vi "Oclaro_FB_INJ_Anritsu.vi"() -> ()   [LabVIEW 2014]
doc: "Use this template to measure or generate signals using the DAQ Assistant Express VI and NI-DAQmx. Double click the DAQ Assistant Express VI to launch a configuration wizard which steps you through configuring a measurement or generation.\n\nNote: You must have an NI-DAQmx compatible device installed to use this Express VI. Refer to the DAQ Quick Start Guide for NI-DAQ 7.0 for a list of compatible devices."
uses:
  Instance           8 18Saved   INJ FB Map .vi
  <instrlib>/Tektronix 7000 Series/Public/Data/Read (Single Waveform).vi
  <instrlib>/Tektronix 7000 Series/Tektronix 7000 Series.lvlib
panel:
  in  "Capture OSA?":bool=TRUE
  in  "Scope Model":string="Tektronix MSO 71254"
  in  "OSA Model":string="Anritsu MS9710C"
  out "Current Source":string="PROFILE-ITC510"
  in  "Resistance (k Ohms)":dbl=10.0
  in  "Time Series Length":dbl=500000.0
  in  "OSA Address":refnum<visa-resource-name>="GPIB0::8::INSTR"
  in  "file path":path=path "Z:/Toomey/Experimental Data/Bangor DFB/2015-07-10/Run01/Data"
  in  "Tek Scope Address":refnum<visa-resource-name>="GPIB0::4::INSTR"
  out "Start time":timestamp=timestamp(3519349015.1862907 s since 1904-01-01)
  in  "Current Source Address":refnum<visa-resource-name>="GPIB0::10::INSTR"
  in  "Channel (0: Channel 1)":u16(ring) format="%#_5f" items=["Channel 1", "Channel 2", "Channel 3", "Channel 4", "Math 1", "Math 2", "Math 3", "Math 4", "Reference 1", "Reference 2", "Reference 3", "Reference 4"]
  out "Current FB":dbl=0.9
  out "Current INJ":dbl=80.0
  in  "Initial Current (mA)":dbl=25.0
  in  "Step Size (mA)":dbl=0.5
  in  "Max Current (mA)":dbl=80.0
  in  "AOM Step":dbl=0.005
  in  "AOM Finish":dbl=0.9
  in  "AOM Start":dbl=0.1
  out "Total Time (hrs)":dbl=47.11827769252989
  out "Finish time":timestamp=timestamp(3519518640.985984 s since 1904-01-01)
  out "INJ (%)":dbl=99.09909909909909
  out "FB (%)":dbl=99.37888198757764
  in  "Time to wait for TEC (sec)":dbl=15.0 caption="Delay Time (s)"
  # "Settings"
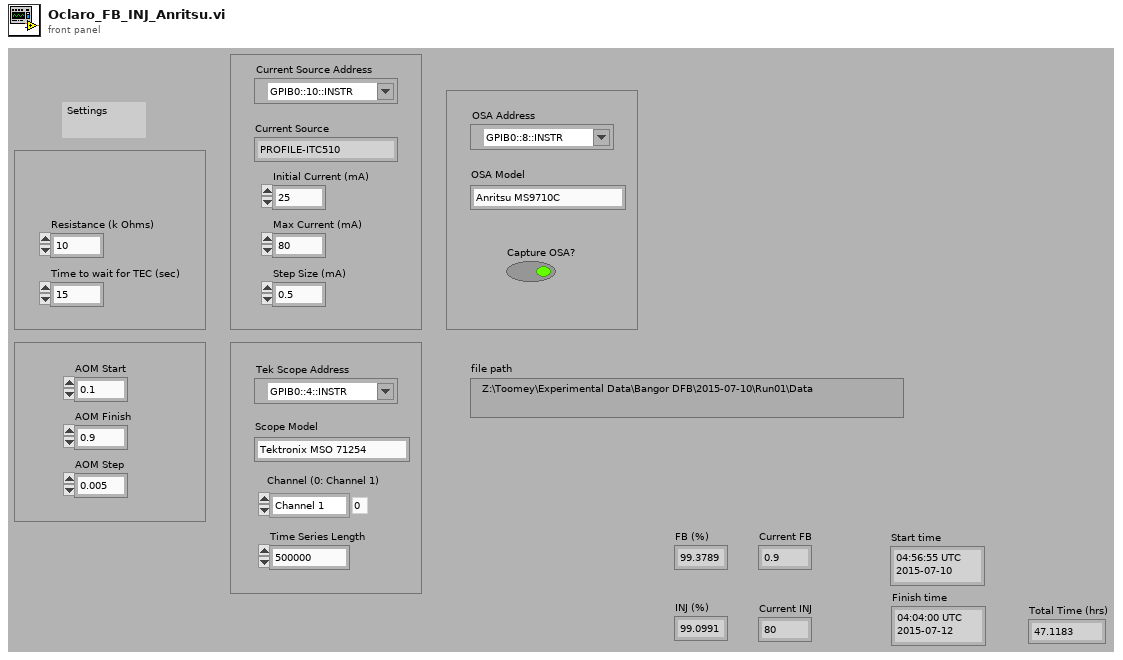
[diagram p1: front panel]
types:
  T1 = cluster{"Start Wavelength(nm)":dbl, "Stop Wavelength(nm)":dbl, "Sampling Points":i32}
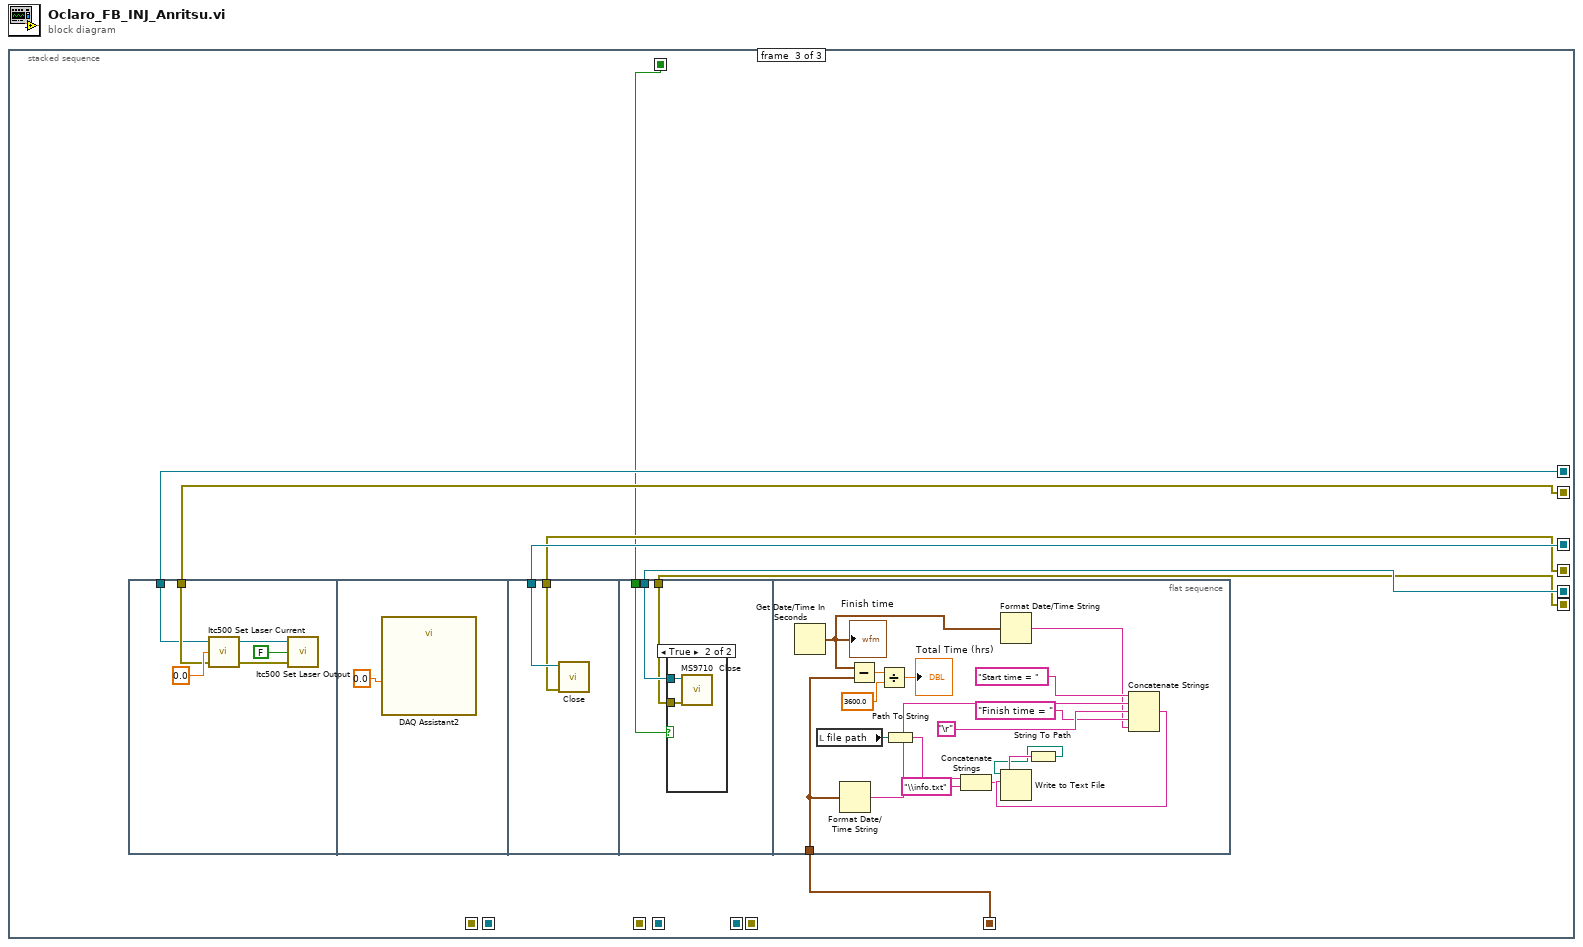
[diagram p0: block diagram]
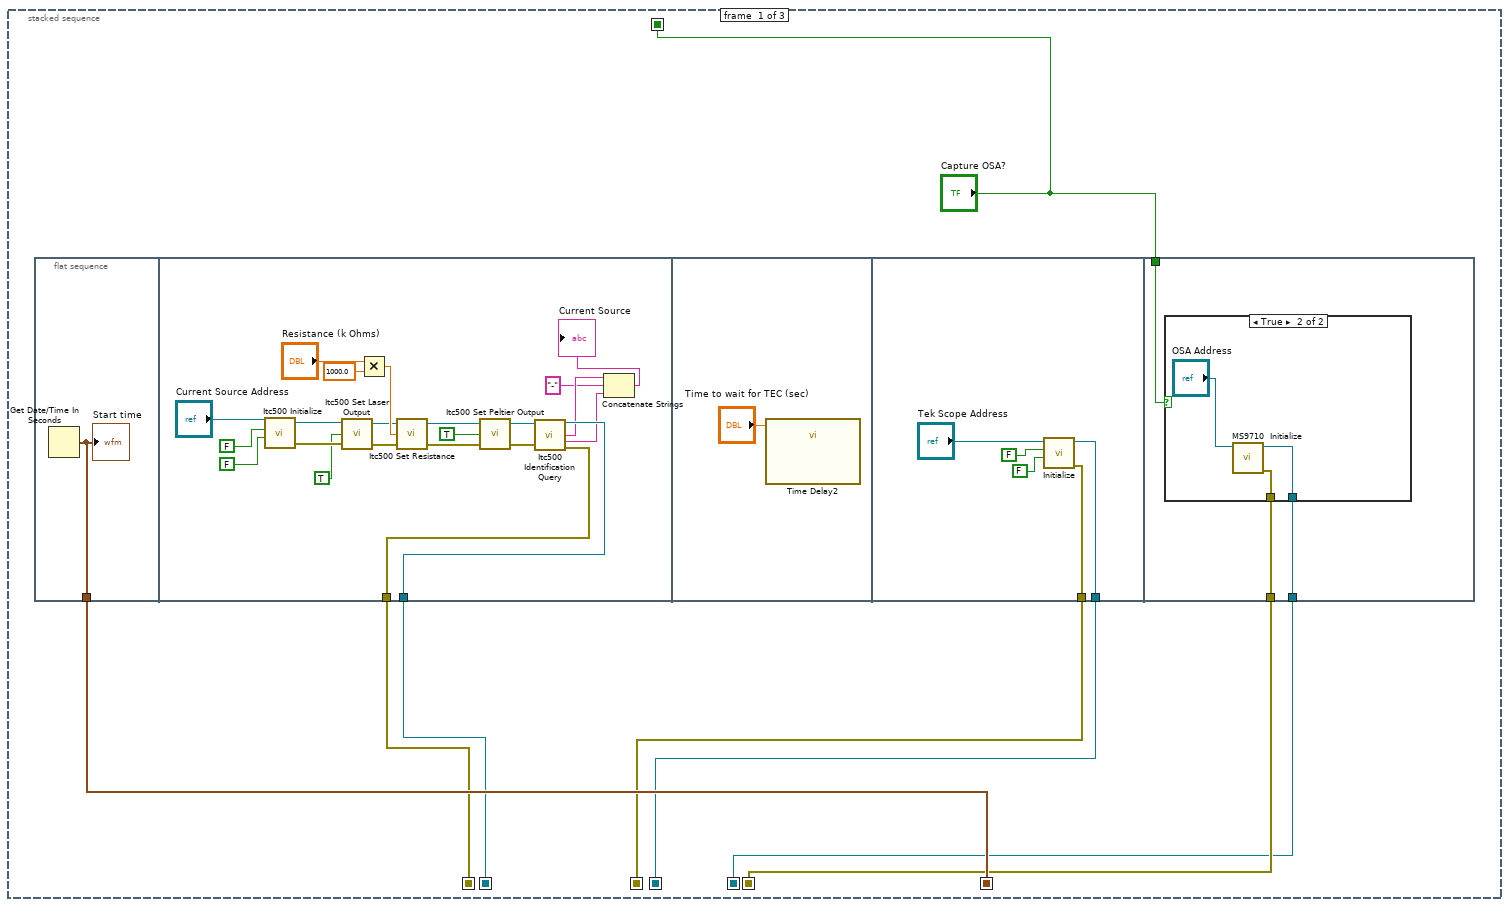
[diagram p2: hidden frame]
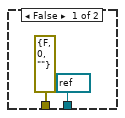
[diagram p3: hidden frame]
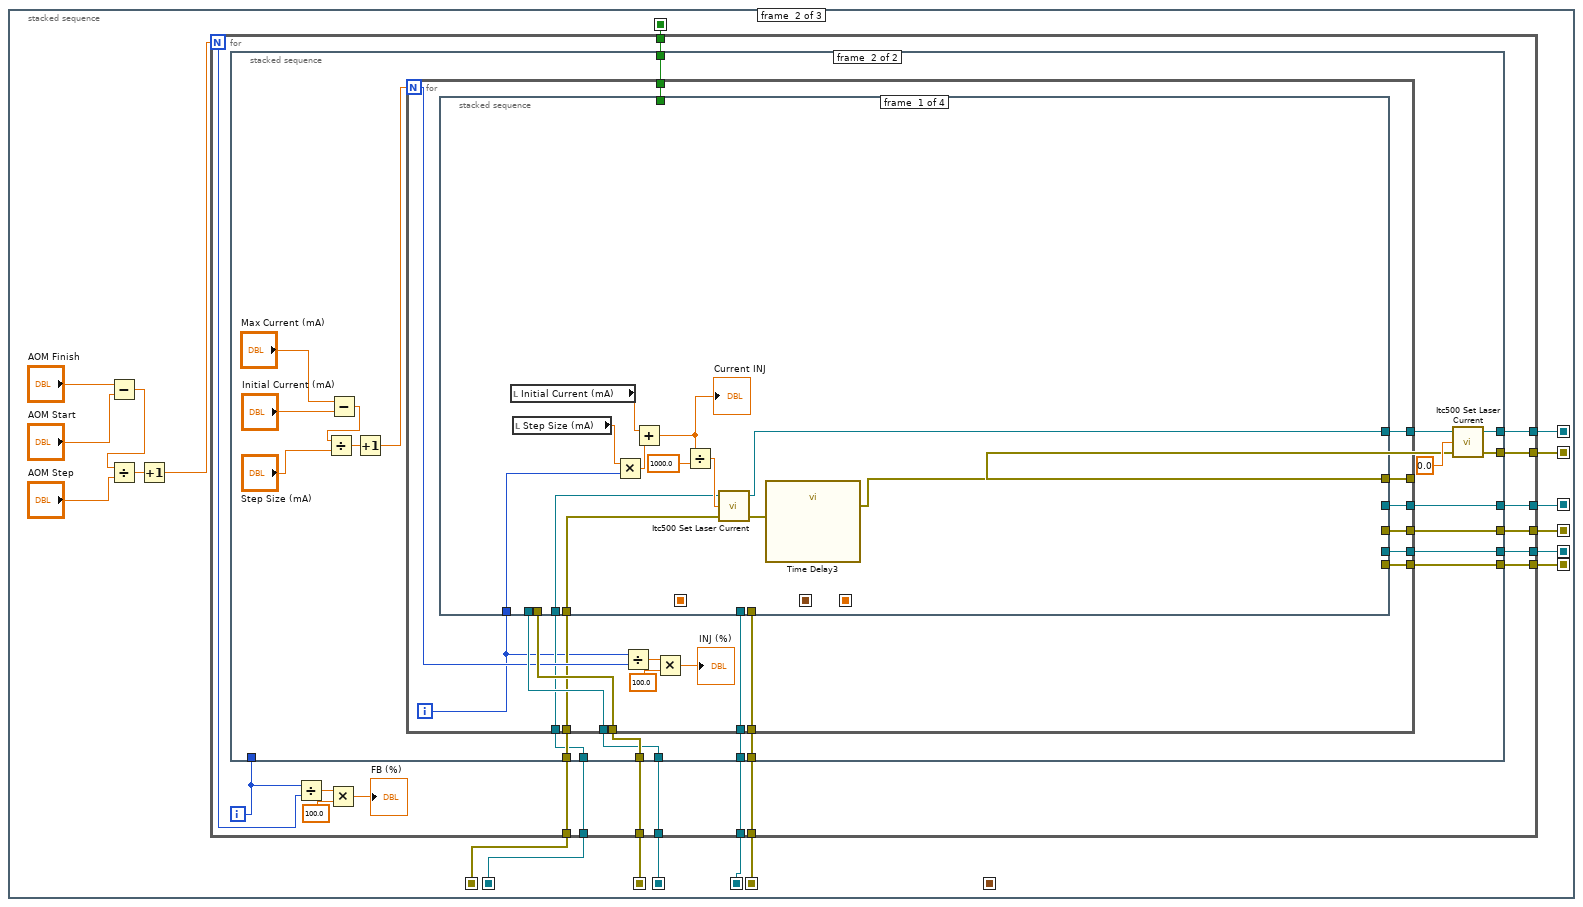
[diagram p4: hidden frame]
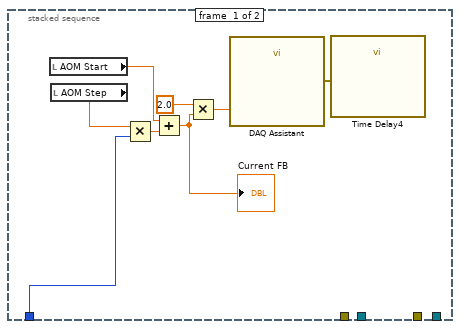
[diagram p5: hidden frame]
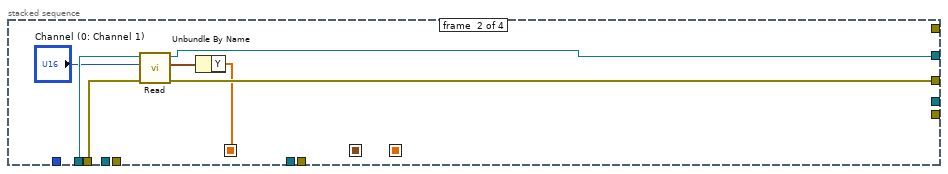
[diagram p6: hidden frame]
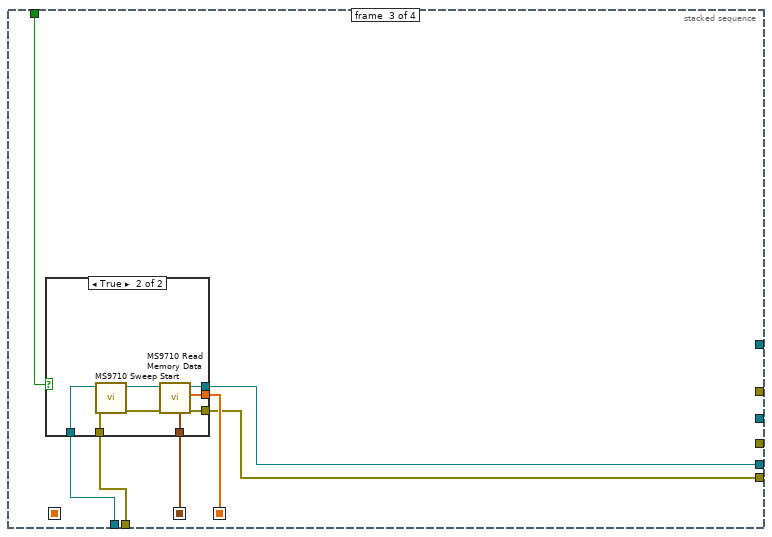
[diagram p7: hidden frame]
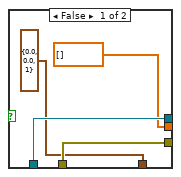
[diagram p8: hidden frame]
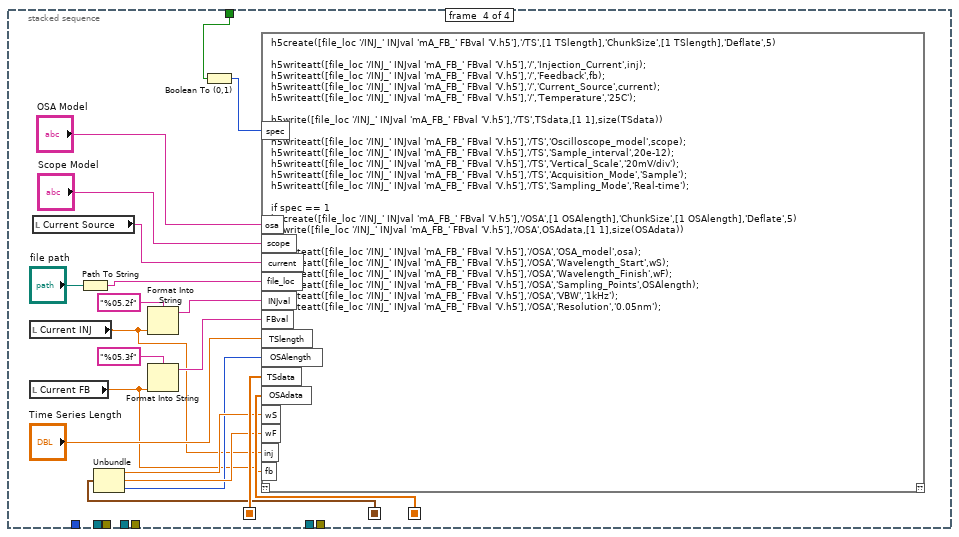
[diagram p9: hidden frame]
diagram:
  n1 = stacked-sequence {
    seq-local: [w5 _ _] -> [_ w62 _]
    seq-local: [w4 _ _] -> [_ w61 _]
    seq-local: [_ w60 _] -> [_ _ w195]
    seq-local: [_ w59 _] -> [_ _ w196]
    seq-local: [w8 _ _] -> [_ _ w192]
    seq-local: [_ w57 _] -> [_ _ w194]
    seq-local: [_ w56 _] -> [_ _ w193]
    seq-local: [w6 _ _] -> [_ w51 _]
    seq-local: [w7 _ _] -> [_ w52 _]
    seq-local: [w2 _ _] -> [_ w50 _]
    seq-local: [w3 _ _] -> [_ w49 _]
    seq-local: [_ w48 _] -> [_ _ w191]
    seq-local: [_ w47 _] -> [_ _ w190]
    seq-local: ["Capture OSA?" _ _] -> [_ w46 w189]
    frame #0 {
      n2 = flat-sequence {
        tunnel: [w9] -> w8
        tunnel: [w15] -> w7
        tunnel: [w14] -> w6
        tunnel: [w34] -> w5
        tunnel: [w33] -> w4
        tunnel: [w40] -> w3
        tunnel: [w39] -> w2
        tunnel: "Capture OSA?" -> [w38]
        frame #0 {
          n3 = Get Date/Time In Seconds() -> (seconds since 1Jan1904=w9:timestamp)
          "Start time" <- w9
        }
        frame #1 {
          n4 = call <instrlib>:"Itc500 Initialize.vi"("reset device"=FALSE, "id query"=FALSE, "resource name"="Current Source Address") -> ("error out"=w31:errorcluster, "instrument handle"=w30:refnum<visa-resource-name>)  [unwired: 1 in, 1 out]
          n5 = call <instrlib>:"Itc500 Set Laser Output.vi"("error in (no error)"=w31, "output"=TRUE, "instrument handle"=w30) -> ("error out"=w19:errorcluster, "instrument handle out"=w18:refnum<visa-resource-name>)  [unwired: 1 out]
          n6 = Multiply(x="Resistance (k Ohms)", y=1000.0) -> (x*y=w25:dbl)
          n7 = call <instrlib>:"Itc500 Set Resistance.vi"("error in (no error)"=w19, "resistance"=w25, "instrument handle"=w18) -> ("error out"=w21:errorcluster, "instrument handle out"=w20:refnum<visa-resource-name>)  [unwired: 1 out]
          n8 = call <instrlib>:"Itc500 Set Peltier Output.vi"("error in (no error)"=w21, "output"=TRUE, "instrument handle"=w20) -> ("error out"=w17:errorcluster, "instrument handle out"=w16:refnum<visa-resource-name>)  [unwired: 1 out]
          n9 = call <instrlib>:"Itc500 Identification Query.vi"("instrument handle"=w16, "error in (no error)"=w17) -> ("instrument handle out"=w14:refnum<visa-resource-name>, "manufacturer name"=w13:string, "instrument name"=w12:string, "error out"=w15:errorcluster)  [unwired: 7 in, 3 out]
          n10 = Concatenate Strings(w13, "-" ("string"), w12) -> (→"Current Source":string)
        }
        frame #2 {
          n11 = call "Time Delay2"("Delay Time (s)"="Time to wait for TEC (sec)") -> ()  [unwired: 10 in, 1 out]
        }
        frame #3 {
          n12 = call <instrlib>:"Initialize.vi"("Reset? ( Yes)"=FALSE ("Reset (T: Reset)"), "ID Query? ( Yes)"=FALSE ("Reset (T: Reset)"), "VISA resource name"="Tek Scope Address") -> ("error out"=w34:errorcluster, "VISA resource name out"=w33:refnum<visa-resource-name>)  [unwired: 7 in]
        }
        frame #4 {
          n13 = case shown="True" w38 {
            tunnel: [errorcluster {"status"=FALSE, "code"=0, "source"=""} ("error out") w44] -> w40
            tunnel: [refnum<visa-resource-name> refnum ("instr handle out") w43] -> w39
            frame False {
            }
            frame True {
              n14 = call <instrlib>:"MS9710  Initialize.vi"("VISA in"="OSA Address") -> ("error out"=w44:errorcluster, "instr handle out"=w43:refnum<visa-resource-name>)  [unwired: 9 in]
            }
          }
        }
      }
    }
    frame #1 {
      n15 = Subtract(x="AOM Finish", y="AOM Start") -> (x-y=w63:dbl)
      n16 = Divide(x=w63, y="AOM Step") -> (x/y=w64:dbl)
      n17 = Increment(x=w64) -> (x+1=w58:dbl)
      n18 = for {
        N: w58 -> [w75]
        tunnel: w51 -> [w82]
        tunnel: w52 -> [w81]
        tunnel: w62 -> [w80]
        tunnel: w61 -> [w79]
        tunnel: [w78] -> w60
        tunnel: [w77] -> w59
        tunnel: [w71] -> w57
        tunnel: [w70] -> w56
        tunnel: w50 -> [w69]
        tunnel: w49 -> [w68]
        tunnel: [w67] -> w48
        tunnel: [w66] -> w47
        tunnel: w46 -> [w65]
        i -> [w76]
        n19 = stacked-sequence {
          tunnel: w82 -> [_ w100]
          tunnel: w81 -> [_ w101]
          tunnel: w76 -> [w90 _]
          tunnel: w80 -> [_ w112]
          tunnel: w79 -> [_ w111]
          tunnel: [_ w97] -> w78
          tunnel: [_ w96] -> w77
          tunnel: [_ w107] -> w71
          tunnel: [_ w106] -> w70
          tunnel: w69 -> [_ w95]
          tunnel: w68 -> [_ w94]
          tunnel: [_ w93] -> w67
          tunnel: [_ w92] -> w66
          tunnel: w65 -> [_ w91]
          frame #0 {
            n20 = local read "AOM Start"() -> (w85:dbl)
            n21 = local read "AOM Step"() -> (w86:dbl)
            n22 = Multiply(x=w86, y=w90) -> (x*y=w89:dbl)
            n23 = Add(x=w85, y=w89) -> (x+y=w88:dbl)
            "Current FB" <- w88
            n24 = Multiply(x=2.0, y=w88) -> (x*y=w87:dbl)
            n25 = call "DAQ Assistant"("data"=w87) -> ("error out"=w84:errorcluster)  [unwired: 17 in, 1 out]
            n26 = call "Time Delay4"("error in (no error)"=w84) -> ()  [unwired: 10 in, 1 out]
          }
          frame #1 {
            n27 = Subtract(x="Max Current (mA)", y="Initial Current (mA)") -> (x-y=w109:dbl)
            n28 = Divide(x=w109, y="Step Size (mA)") -> (x/y=w110:dbl)
            n29 = Increment(x=w110) -> (x+1=w108:dbl)
            n30 = for {
              N: w108 -> [w124]
              tunnel: [w130] -> w99
              tunnel: w112 -> [w129]
              tunnel: w111 -> [w128]
              tunnel: [w123] -> w107
              tunnel: [w122] -> w106
              tunnel: w101 -> [w121]
              tunnel: w100 -> [w120]
              tunnel: [w119] -> w98
              tunnel: w95 -> [w117]
              tunnel: w94 -> [w116]
              tunnel: [w115] -> w93
              tunnel: [w114] -> w92
              tunnel: w91 -> [w113]
              i -> [w118]
              n31 = stacked-sequence {
                seq-local: [_ w143 _ _] -> [_ _ _ w186]
                seq-local: [_ _ w156 _] -> [_ _ _ w185]
                seq-local: [_ _ w155 _] -> [_ _ _ w184]
                tunnel: w118 -> [w136 _ _ _]
                tunnel: [w133 _ _ _] -> w130
                tunnel: w129 -> [_ w148 _ _]
                tunnel: w128 -> [_ w149 _ _]
                tunnel: [_ w146 _ _] -> w123
                tunnel: [_ w144 _ _] -> w122
                tunnel: w121 -> [w135 _ _ _]
                tunnel: w120 -> [w134 _ _ _]
                tunnel: [w132 _ _ _] -> w119
                tunnel: w117 -> [_ _ w154 _]
                tunnel: w116 -> [_ _ w153 _]
                tunnel: [_ _ w152 _] -> w115
                tunnel: [_ _ w151 _] -> w114
                tunnel: w113 -> [_ _ w150 w170]
                frame #0 {
                  n32 = local read "Initial Current (mA)"() -> (w138:dbl)
                  n33 = local read "Step Size (mA)"() -> (w137:dbl)
                  n34 = Multiply(x=w137, y=w136) -> (x*y=w141:dbl)
                  n35 = Add(x=w138, y=w141) -> (x+y=w131:dbl)
                  "Current INJ" <- w131
                  n36 = Divide(x=w131, y=1000.0) -> (x/y=w139:dbl)
                  n37 = call <instrlib>:"Itc500 Set Laser Current.vi"("error in (no error)"=w135, "current"=w139, "instrument handle"=w134) -> ("error out"=w140:errorcluster, "instrument handle out"=w132:refnum<visa-resource-name>)  [unwired: 1 out]
                  n38 = call "Time Delay3"("error in (no error)"=w140) -> ("error out"=w133:errorcluster)  [unwired: 10 in]
                }
                frame #1 {
                  n39 = call-poly <instrlib>:"Read.vi"("error in (no error)"=w148, "Channel (0: Channel 1)"="Channel (0: Channel 1)", "VISA resource name"=w149) -> ("error out"=w144:errorcluster, "Waveform Data"=w147:waveform(dbl), "VISA resource name out"=w146:refnum<visa-resource-name>)  [unwired: 6 in]
                  n40 = Unbundle By Name(w147) -> ("Y"=w143:dbl[])
                }
                frame #2 {
                  n41 = case shown="True" w150 {
                    tunnel: [dbl[] [] ("Data") w166] -> w156
                    tunnel: [T1 {"Start Wavelength(nm)"=0.0, "Stop Wavelength(nm)"=0.0, "Sampling Points"=1} ("Condition Data") w165] -> w155
                    tunnel: w154 -> [w159 w164]
                    tunnel: w153 -> [w160 w163]
                    tunnel: [w159 w162] -> w152
                    tunnel: [w160 w161] -> w151
                    frame False {
                    }
                    frame True {
                      n42 = call <instrlib>:"MS9710 Sweep Start.vi"("error in (no error)"=w163, "instr handle in"=w164) -> ("error out"=w168:errorcluster, "instr handle out"=w167:refnum<visa-resource-name>)  [unwired: 8 in]
                      n43 = call <instrlib>:"MS9710 Read Memory Data.vi"("error in (no error)"=w168, "instr handle in"=w167) -> ("error out"=w161:errorcluster, "Data"=w166:dbl[], "instr handle out"=w162:refnum<visa-resource-name>, "Condition Data"=w165:T1)  [unwired: 5 in, 1 out]
                    }
                  }
                }
                frame #3 {
                  n44 = local read "Current INJ"() -> (w171:dbl)
                  n45 = local read "Current FB"() -> (w172:dbl)
                  n46 = local read "Current Source"() -> (w175:string)
                  n47 = Path To String(path="file path") -> (string=w188:string)
                  n48 = Unbundle(w184) -> ("Start Wavelength(nm)"=w183:dbl, "Stop Wavelength(nm)"=w182:dbl, "Sampling Points"=w180:i32)
                  n49 = Format Into String(format string="%05.2f", w171) -> (resulting string=w179:string)  [unwired: 2 in, 1 out]
                  n50 = Format Into String(format string="%05.3f", w172) -> (resulting string=w181:string)  [unwired: 2 in, 1 out]
                  n51 = Boolean To (0,1)(Boolean=w170) -> (0, 1=w169:i16)
                  n52 = script code="h5create([file_loc '/INJ_' INJval 'mA_FB_' FBval 'V.h5'],'/TS',[1 TSlength],'ChunkSize',[1 TSlength],'Deflate',5)\n\nh5writeatt([file_loc '/INJ_' INJval 'mA_FB_' FBval 'V.h5'],'/','Injection_Current',inj);\nh5writeatt([file_loc '/INJ_' INJval 'mA_FB_' FBval 'V.h5'],'/','Feedback',fb);\nh5writeatt([file_loc '/INJ_' INJval 'mA_FB_' FBval 'V.h5'],'/','Current_Source',current);\nh5writeatt([file_loc '/INJ_' INJval 'mA_FB_' FBval 'V.h5'],'/','Temperature','25C');\n\nh5write([file_loc '/INJ_' INJval 'mA_FB_' FBval 'V.h5'],'/TS',TSdata,[1 1],size(TSdata))\n\nh5writeatt([file_loc '/INJ_' INJval 'mA_FB_' FBval 'V.h5'],'/TS','Oscilloscope_model',scope);\nh5writeatt([file_loc '/INJ_' INJval 'mA_FB_' FBval 'V.h5'],'/TS','Sample_interval',20e-12);\nh5writeatt([file_loc '/INJ_' INJval 'mA_FB_' FBval 'V.h5'],'/TS','Vertical_Scale','20mV/div');\nh5writeatt([file_loc '/INJ_' INJval 'mA_FB_' FBval 'V.h5'],'/TS','Acquisition_Mode','Sample');\nh5writeatt([file_loc '/INJ_' INJval 'mA_FB_' FBval 'V.h5'],'/TS','Sampling_Mode','Real-time');\n\nif spec == 1\nh5create([file_loc '/INJ_' INJval 'mA_FB_' FBval 'V.h5'],'/OSA',[1 OSAlength],'ChunkSize',[1 OSAlength],'Deflate',5)\nh5write([file_loc '/INJ_' INJval 'mA_FB_' FBval 'V.h5'],'/OSA',OSAdata,[1 1],size(OSAdata))\n\nh5writeatt([file_loc '/INJ_' INJval 'mA_FB_' FBval 'V.h5'],'/OSA','OSA_model',osa);\nh5writeatt([file_loc '/INJ_' INJval 'mA_FB_' FBval 'V.h5'],'/OSA','Wavelength_Start',wS);\nh5writeatt([file_loc '/INJ_' INJval 'mA_FB_' FBval 'V.h5'],'/OSA','Wavelength_Finish',wF);\nh5writeatt([file_loc '/INJ_' INJval 'mA_FB_' FBval 'V.h5'],'/OSA','Sampling_Points',OSAlength);\nh5writeatt([file_loc '/INJ_' INJval 'mA_FB_' FBval 'V.h5'],'/OSA','VBW','1kHz');\nh5writeatt([file_loc '/INJ_' INJval 'mA_FB_' FBval 'V.h5'],'/OSA','Resolution','0.05nm');\nend"("file_loc"=w188, "INJval"=w179, "FBval"=w181, "TSlength"="Time Series Length", "OSAlength"=w180, "TSdata"=w186, "OSAdata"=w185, "wS"=w183, "wF"=w182, "inj"=w171, "fb"=w172, "current"=w175, "scope"="Scope Model", "osa"="OSA Model", "spec"=w169) -> ()  [unwired: 1 in, 1 out]
                }
              }
              n53 = Divide(x=w118, y=w124) -> (x/y=w127:dbl)
              n54 = Multiply(x=w127, y=100.0) -> (x*y=→"INJ (%)":dbl)
            }
            n55 = call <instrlib>:"Itc500 Set Laser Current.vi"("error in (no error)"=w99, "current"=0.0, "instrument handle"=w98) -> ("error out"=w96:errorcluster, "instrument handle out"=w97:refnum<visa-resource-name>)  [unwired: 1 out]
          }
        }
        n56 = Divide(x=w76, y=w75) -> (x/y=w74:dbl)
        n57 = Multiply(x=w74, y=100.0) -> (x*y=→"FB (%)":dbl)
      }
    }
    frame #2 {
      n58 = flat-sequence {
        tunnel: w196 -> [w198]
        tunnel: w195 -> [w197]
        tunnel: w194 -> [w205]
        tunnel: w193 -> [w204]
        tunnel: w191 -> [w208]
        tunnel: w190 -> [w207]
        tunnel: w189 -> [w206]
        tunnel: w192 -> [w222]
        frame #0 {
          n59 = call <instrlib>:"Itc500 Set Laser Current.vi"("error in (no error)"=w198, "current"=0.0, "instrument handle"=w197) -> ("error out"=w201:errorcluster, "instrument handle out"=w200:refnum<visa-resource-name>)  [unwired: 1 out]
          n60 = call <instrlib>:"Itc500 Set Laser Output.vi"("error in (no error)"=w201, "output"=FALSE, "instrument handle"=w200) -> ()  [unwired: 3 out]
        }
        frame #1 {
          n61 = call "DAQ Assistant2"("data"=0.0) -> ()  [unwired: 17 in, 2 out]
        }
        frame #2 {
          n62 = call <instrlib>:"Close.vi"("error in (no error)"=w204, "VISA resource name"=w205) -> ()  [unwired: 9 in, 1 out]
        }
        frame #3 {
          n63 = case shown="True" w206 {
            tunnel: w208 -> [_ w210]
            tunnel: w207 -> [_ w209]
            frame False {
            }
            frame True {
              n64 = call <instrlib>:"MS9710  Close.vi"("error in (no error)"=w209, "instr handle in"=w210) -> ()  [unwired: 9 in, 1 out]
            }
          }
        }
        frame #4 {
          n65 = Get Date/Time In Seconds() -> (seconds since 1Jan1904=w220:timestamp)
          "Finish time" <- w220
          n66 = local read "file path"() -> (w215:path)
          n67 = Format Date/Time String(seconds (now)=w222) -> (date/time string=w221:string)  [unwired: 2 in]
          n68 = Subtract(x=w220, y=w222) -> (x-y=w225:dbl)
          n69 = Divide(x=w225, y=3600.0) -> (x/y=→"Total Time (hrs)":dbl)
          n70 = Path To String(path=w215) -> (string=w212:string)
          n71 = Concatenate Strings(w212, "\\info.txt" ("string")) -> (w214:string)
          n72 = Format Date/Time String(seconds (now)=w220) -> (date/time string=w217:string)  [unwired: 2 in]
          n73 = String To Path(string=w214) -> (path=w213:path)
          n74 = Concatenate Strings("Start time = ", w221, "\r", "Finish time = ", w217) -> (w216:string)
          n75 = Write to Text File(file (use dialog)=w213, text=w216) -> ()  [unwired: 2 in, 3 out]
        }
      }
    }
  }
